vi "NILIA_PLL_Locked.vi"(11 "f":fxp<+/-,32,0> format="%.32g") -> (3 "locked":bool)   [LabVIEW 2012]
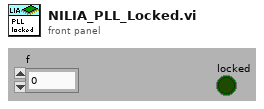
[diagram p1: front panel]
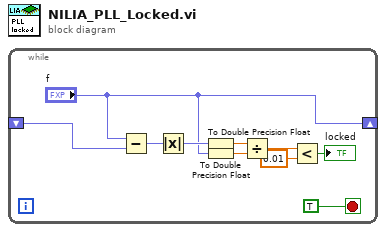
[diagram p0: block diagram]
diagram:
  n1 = while {
    shift-right: ["f"] -> _
    shift-left: _ -> [w10]
    stop <- TRUE stop-if-true
    n2 = Subtract(x="f", y=w10) -> (x-y=w9:fxp<+/-,33,1>)
    n3 = Absolute Value(x=w9) -> (abs(x)=w8:fxp<+,32,0>)
    n4 = To Double Precision Float(number=w8) -> (double precision float=w7:dbl)
    n5 = To Double Precision Float(number="f") -> (double precision float=w6:dbl)
    n6 = Divide(x=w7, y=w6) -> (x/y=w4:dbl)
    n7 = Less?(x=w4, y=0.01) -> (x < y?=→"locked":bool)
  }
